vi "Measure.vi"(8 "error in":errorcluster, 11 "UDP in":refnum<class "UDP.lvclass">) -> (0 "error out":errorcluster, 2 "Measurement Results":T1={"Voltage (V)"=1.0} {"Voltage (V)" min=-424.2 max=424.2 step=1.0 format="%#.1f"}, 3 "UDP out":refnum<class "UDP.lvclass">)   [LabVIEW 2020, in "Plugin Instrument Driver.lvlib" / "UDP.lvclass"]
doc: "Read Measurement."
uses:
  UDP.lvclass
  C:/SVN_LabSys/labsys_lvcode/LabSys_SourceCode/Plugin Template/Source/Drivers/Instrument Driver/Instrument Driver.lvclass
  Typedefs/Measurement Results.ctl
  Typedefs/Device Details.ctl
  Instrument Driver.lvclass
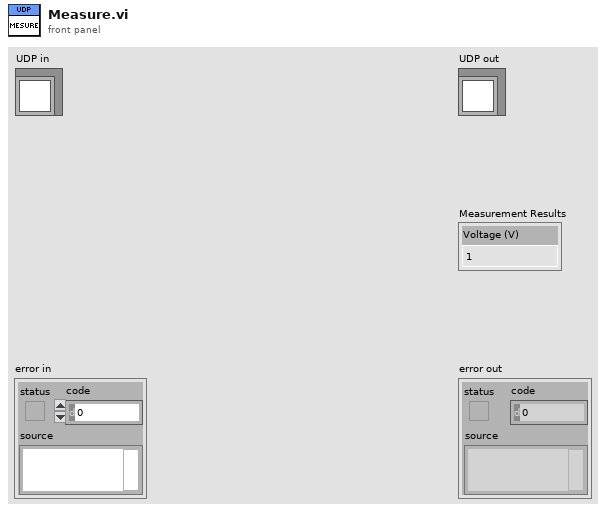
[diagram p1: front panel]
types:
  T1 = typedef "Plugin Instrument Driver.lvlib/Instrument Driver.lvclass/Measurement Results.ctl" = cluster{"Voltage (V)":dbl}
  T2 = typedef "Plugin Instrument Driver.lvlib/UDP.lvclass/Device Details.ctl" = cluster{"Device Port Number":u16, "Device IP":string, "Timeout":i32, "Port Number":u16, "Connection ID":refnum<k16>}
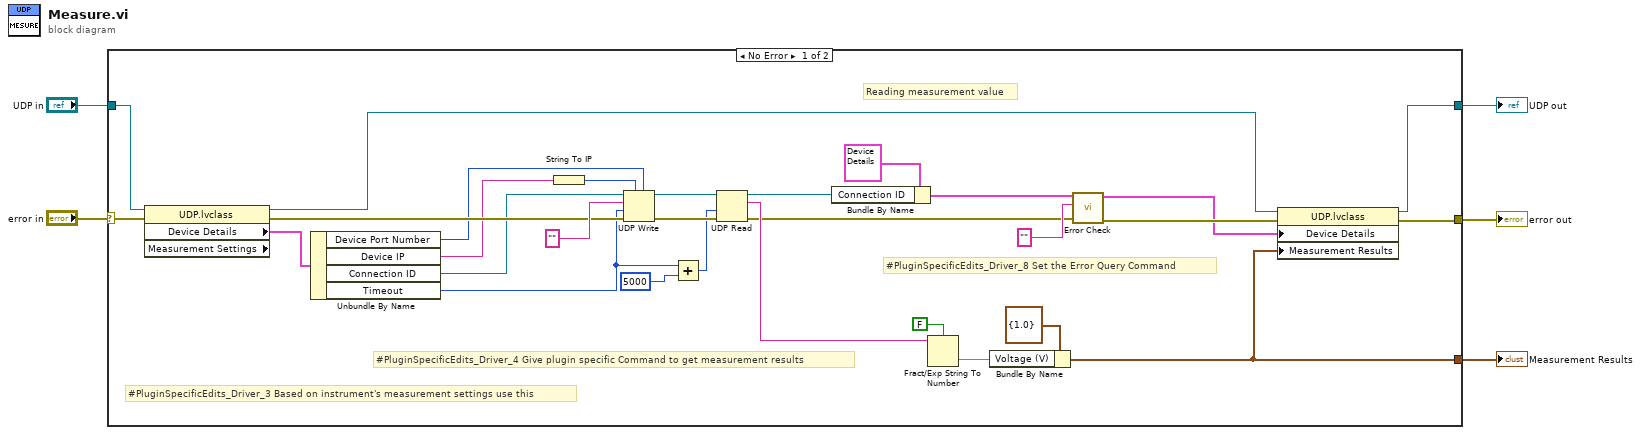
[diagram p0: block diagram]
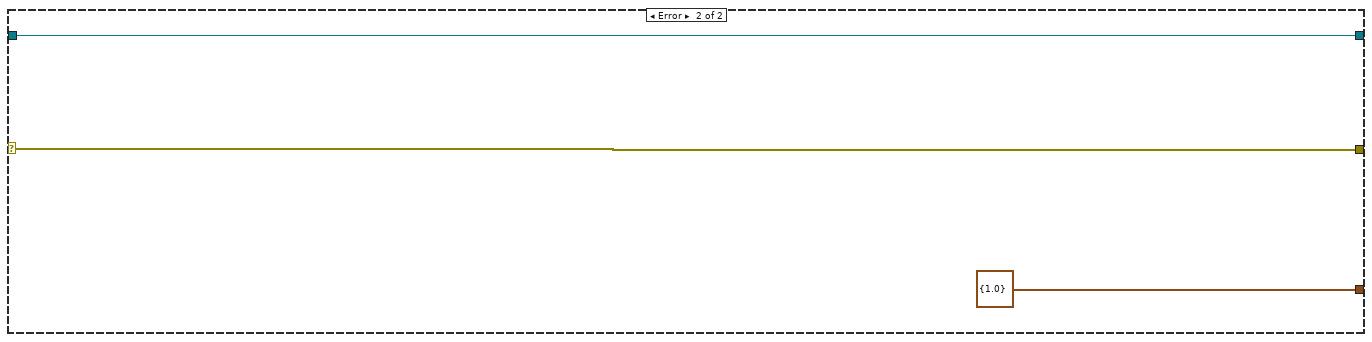
[diagram p2: hidden frame]
diagram:
  n1 = case shown="No Error" "error in" {
    selector: "error in" -> [w29 w36]
    tunnel: "UDP in" -> [w30 w37]
    tunnel: [w26 w37] -> w3
    tunnel: [w25 w36] -> w2
    tunnel: [w12 T1 {"Voltage (V)"=1.0} ("Measurement Results")] -> w1
    frame No Error {
      # "#PluginSpecificEdits_Driver_3 Based on instrument's measurement settings use this"
      # "#PluginSpecificEdits_Driver_8 Set the Error Query Command"
      # "#PluginSpecificEdits_Driver_4 Give plugin specific Command to get measurement results"
      # "Reading measurement value"
      n2 = property class="UDP.lvclass" props=["Device Details", "Measurement Settings"](reference=w30, error in=w29) -> (reference out=w27:refnum<class "UDP.lvclass">, error out=w28:errorcluster, "Device Details"=w22:T2)  [unwired: 1 out]
      n3 = Unbundle By Name(w22) -> ("Device Port Number"=w21:u16, "Device IP"=w20:string, "Connection ID"=w19:refnum<k16>, "Timeout"=w18:i32)
      n4 = String To IP(1:w20) -> (0:w34:u32)
      n5 = UDP Write(address=w34, port or service name=w21, connection ID=w19, data in="", 8:w28, 9:w18) -> (error out=w32:errorcluster, 3:w23:refnum<k16>)
      n6 = Add(x=w18, y=5000) -> (x+y=w24:i32)
      n7 = UDP Read(connection ID=w23, timeout ms (25000)=w24, 8:w32) -> (data out=w15:string, error out=w6:errorcluster, 3:w16:refnum<k16>)  [unwired: 1 in, 2 out]
      n8 = Bundle By Name(cluster=T2 {"Device Port Number"=2001, "Device IP"="192.168.1.1.100", "Timeout"=5000, "Port Number"=1234, "Connection ID"=refnum} ("Device Details"), "Connection ID"=w16) -> (w10:T2)
      n9 = Fract/Exp String To Number(use system decimal point (T)=FALSE, string=w15) -> (number=w13:dbl)  [unwired: 2 in, 1 out]
      n10 = Bundle By Name(cluster=T1 {"Voltage (V)"=1.0} ("Measurement Results"), "Voltage (V)"=w13) -> (w12:T1)
      n11 = call "Error Check.vi"("error in"=w6, "Error Query Command"="" ("data in"), "Device Details in"=w10) -> ("error out"=w9:errorcluster, "Device Details out"=w8:T2)  [unwired: 7 in]
      n12 = property class="UDP.lvclass"(reference=w27, error in=w9, "Device Details"=w8, "Measurement Results"=w12) -> (reference out=w26:refnum<class "UDP.lvclass">, error out=w25:errorcluster)
    }
    frame Error {
    }
  }
  "error out" <- w2
  "UDP out" <- w3
  "Measurement Results" <- w1
